vi "ReadWrite.Data.ForceWrite.vi"(8 "error in (no error)":errorcluster, 11 "Ref":T1) -> (0 "error out":errorcluster)   [LabVIEW 2024, in "Data Access Engine.lvlib" / "Data Access Engine.lvclass"]
uses:
  Data Access Engine.lvclass
  Data Access Engine.lvclass/Data Access Engine.ctl
  Access Type Classes/ReadWrite/ReadWrite.lvclass
  Types/ReadWrite.DVR.ctl
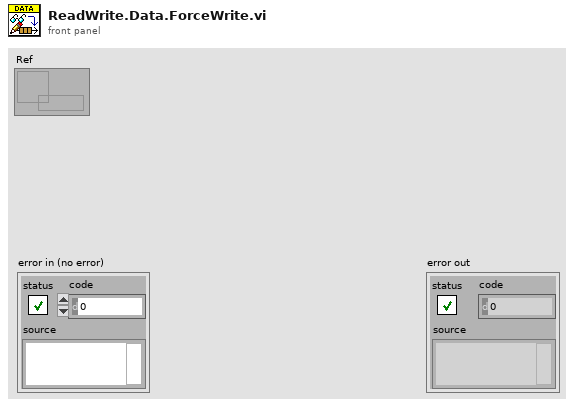
[diagram p1: front panel]
types:
  T1 = typedef "Data Access Engine.lvlib/Data Access Engine.lvclass/ReadWrite.DVR.ctl" = refnum<data-value>
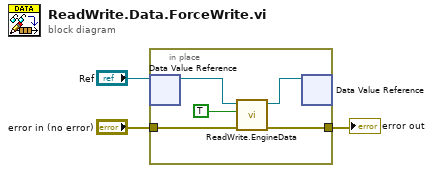
[diagram p0: block diagram]
diagram:
  n1 = in-place {
    in-place-border: "error in (no error)" -> [w8]
    in-place-border: [w7] -> w1
    n2 = in-place-dvr #1("Ref") -> (w6:refnum<class "ReadWrite.lvclass">)  [unwired: 1 out]
    n3 = call "ReadWrite.EngineData.vi"("error in"=w8, "Force"=TRUE, "ReadWrite in"=w6) -> ("error out"=w7:errorcluster, "ReadWrite out"=w5:refnum<class "ReadWrite.lvclass">)  [unwired: 7 in]
    n4 = in-place-dvr #1(w5) -> ()  [unwired: 2 out]
  }
  "error out" <- w1
